vi "Group ID to Tree Items.vi"(8 "error in (no error)":errorcluster, 9 "Group ID":string, 11 "Application Data in":T2) -> (0 "error out":errorcluster, 1 "Settings":T1, 2 "Item":T1, 3 "Application Data out":T2)   [LabVIEW 2017, in "DSF Configuration Utility.lvlib"]
uses:
  DSF Configuration Utility.lvlib
  Main VI/Application Data.ctl
  DSF Configuration API/1.0.0/Public/Controls/DSF Config Data RefNum.ctl
  Main VI/Window State.ctl
  Main VI/View Mode.ctl
  Tree Item Management/Tree Item.ctl
  Tree Item Type.ctl
  DSF Configuration API/1.0.0/Public/Read Item/Read Group.vi
  DSF Configuration API/1.0.0/Public/Read Item/Read Settings.vi
  DSF Configuration API/1.0.0/DSF Configuration API.lvlib
panel:
  # "App\nData"
  # "App\nData"
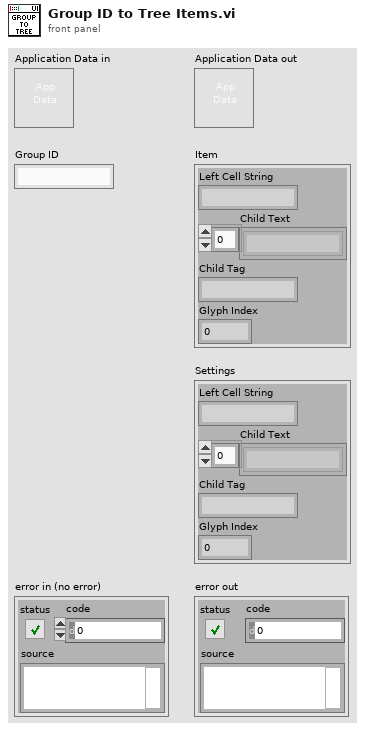
[diagram p1: front panel]
types:
  T1 = typedef "DSF Configuration Utility.lvlib/Tree Item.ctl" = cluster{"Left Cell String":string, "Child Text":string[], "Child Tag":string, "Glyph Index":i32}
  T2 = typedef "DSF Configuration Utility.lvlib/Application Data.ctl" = cluster{"DSF Refnum out":T3, "Tree Control":refnum<vi>, "Tab Control":refnum<vi>, "Top-Level VI":refnum<vi>, "value control refs":refnum<vi>[], "View State":T4}
  T3 = typedef "DSF Configuration API.lvlib/DSF Config Data RefNum.ctl" = refnum<k1>
  T4 = typedef "DSF Configuration Utility.lvlib/View Mode.ctl" = enum16{"Tree", "List"}
  T5 = typedef "DSF Configuration Utility.lvlib/Tree Item Type.ctl" = enum16{"Plugin", "Group", "Transfer", "Channel", "Setting"}
  T6 = typedef "DSF Configuration API.lvlib/DSF Group Info.ctl" = cluster{"direction":i32, "timing":T7, "transfer ids":string[], "settings id":string}
  T7 = typedef "DSF Configuration API.lvlib/DSF Timing Info.ctl" = cluster{"decimation":i32, "offset":i32}
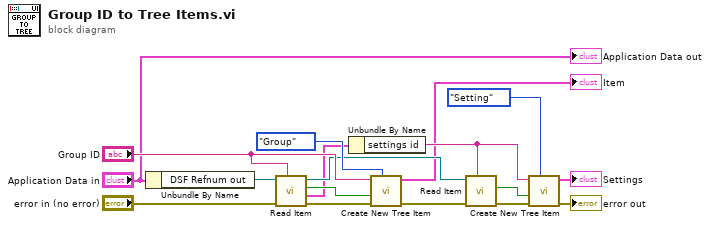
[diagram p0: block diagram]
diagram:
  n1 = Unbundle By Name("Application Data in") -> ("DSF Refnum out"=w3:T3)
  n2 = call-poly "Read Item.vi"("name"="Group ID", "error in (no error)"="error in (no error)", "refnum"=w3) -> ("error out"=w13:errorcluster, "value"=w6:T6, "found?"=w11:bool, "refnum out"=w8:T3)  [unwired: 5 in]
  n3 = Unbundle By Name(w6) -> ("settings id"=w10:string)
  n4 = call "Create New Tree Item.vi"("Item Type"=Tree_Item_Type."Group", "error in"=w13, "found?"=w11, "Left Cell String"="Group ID") -> ("error out"=w14:errorcluster, "Item"=→"Item":T1)  [unwired: 6 in]
  n5 = call-poly "Read Item.vi"("name"=w10, "error in (no error)"=w14, "refnum"=w8) -> ("error out"=w15:errorcluster, "found?"=w12:bool)  [unwired: 5 in, 2 out]
  n6 = call "Create New Tree Item.vi"("Item Type"=Tree_Item_Type."Setting", "error in"=w15, "found?"=w12, "Left Cell String"=w10) -> ("error out"=→"error out":errorcluster, "Item"=→"Settings":T1)  [unwired: 6 in]
  "Application Data out" <- "Application Data in"
